vi "SEA-9811_ReceiverLoopback_FPGA.vi"() -> ()   [LabVIEW 2017]
doc: "This example demonstrates the SEA 9811 loopback mode. Please use the corresponding RT VI to operate this FPGA VI. \n\nCopyright (c) 2013-2019 S.E.A. Datentechnik GmbH, Germany"
uses:
  <vilib>/eio/EIOPropertyNode/EIOPropertyNode.xnode
  <vilib>/rvi/eio/common/nirviEmuTemplateMethod_errors.vi
  <vilib>/rvi/eio/common/nirviEmuTemplatePropertyGet_errors.vi
  <vilib>/rvi/eio/common/nirviEmuTemplatePropertyGet_noerrors.vi
  <vilib>/rvi/eio/common/nirviEmuTemplatePropertySet_errors.vi
  <vilib>/rvi/eio/common/nirviEmuTemplatePropertySet_noerrors.vi
  <vilib>/eio/EIOMethodNode/EIOMethodNode.xnode
  <vilib>/eio/EIONode/EIONode.xnode
panel:
  in  "Rx ConfigData":u16 format="%04x"
  in  "Read Rx Data":bool
  in  "Write Rx SimData":bool
  out "Rx Status Register":u16=255 format="%016b"
  out "CH7":u32 format="%08x"
  out "CH6":u32 format="%08x"
  out "CH5":u32 format="%08x"
  out "CH4":u32 format="%08x"
  out "CH3":u32 format="%08x"
  out "CH2":u32 format="%08x"
  out "CH1":u32 format="%08x"
  out "CH0":u32 format="%08x"
  in  "Rx Sim Data":u32=2271560481 format="%.0x"
  in  "stop":bool
  # "Please refer to VI description for instructions!"
  # "Note: \n\nThe transmitter doesn't send data in the bit order set in the control,\nbut rather changes the bit order when transmitting data. \nThe receiver changes the bit order back before outputting it,\nso that the original bit order is restored and the sent data\nequals the data received.\n\nThe Loopback transmitter DOES NOT change the data when transmitting. Therefore, in this FPGA VI the transmitted data does not equal the data received. Please refer to the real-time VI of this example to see how the data must be reversed to receive the same data at the receiver(s)."
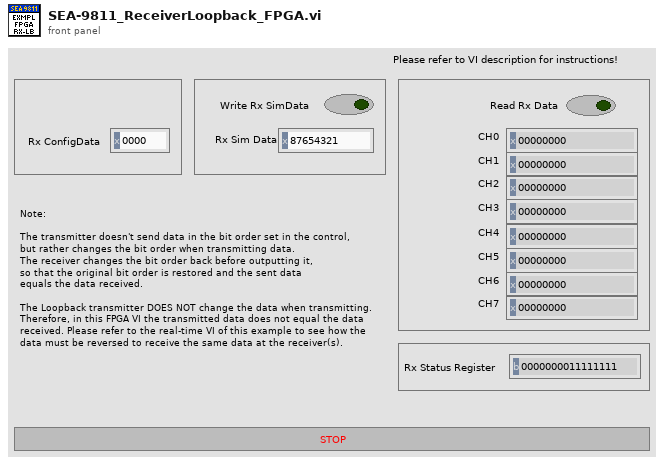
[diagram p1: front panel]
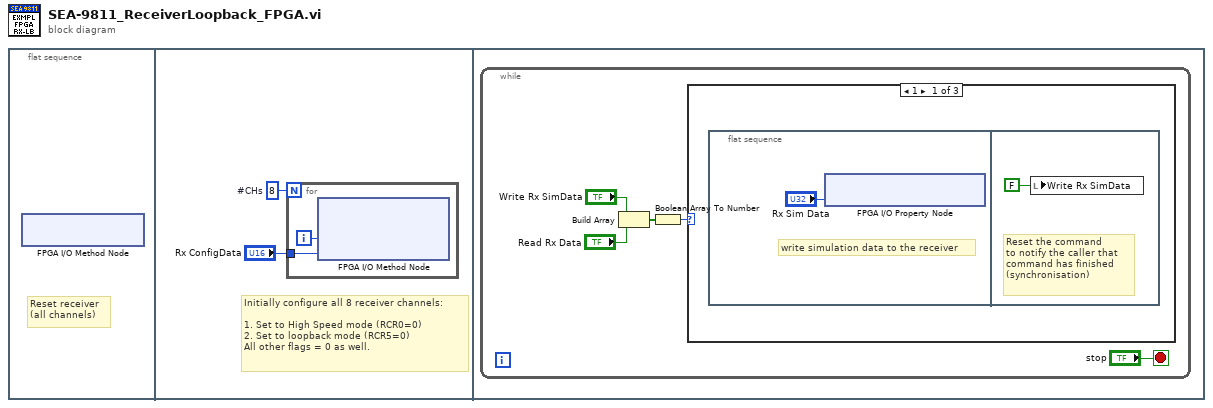
[diagram p0: block diagram]
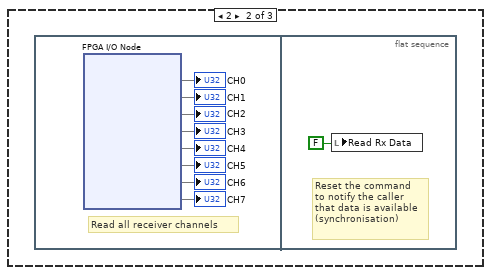
[diagram p2: hidden frame]
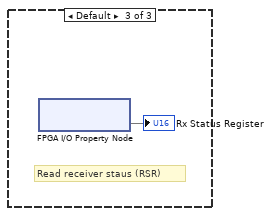
[diagram p3: hidden frame]
diagram:
  n1 = flat-sequence {
    frame #0 {
      # "Reset receiver\n(all channels)"
      n2 = xnode "FPGA I/O Method Node"() -> ()  [unwired: 1 in, 1 out]
    }
    frame #1 {
      w2 = 8  # #CHs
      # "Initially configure all 8 receiver channels: \n\n1. Set to High Speed mode (RCR0=0)\n2. Set to loopback mode (RCR5=0)\nAll other flags = 0 as well."
      n3 = for {
        N: w2 -> [_]
        tunnel: "Rx ConfigData" -> [w4]
        i -> [w3]
        n4 = xnode "FPGA I/O Method Node"("Channel Number"=w3, "Control Register"=w4) -> ()  [unwired: 1 in, 1 out]
      }
    }
    frame #2 {
      n5 = while {
        stop <- "stop" stop-if-true
        n6 = Build Array("Write Rx SimData", "Read Rx Data") -> (w6:bool[])
        n7 = Boolean Array To Number(Boolean array=w6) -> (number=w5:u8)
        n8 = case shown="1" w5 {
          frame 1 {
            n9 = flat-sequence {
              frame #0 {
                # "write simulation data to the receiver"
                n10 = xnode "FPGA I/O Property Node"("Rx SimData HighSpeed"="Rx Sim Data") -> ()  [unwired: 1 in, 1 out]
              }
              frame #1 {
                # "Reset the command\nto notify the caller that\ncommand has finished\n(synchronisation)"
                n11 = local write "Write Rx SimData"(FALSE ("Write SimData")) -> ()
              }
            }
          }
          frame 2 {
            n12 = flat-sequence {
              frame #0 {
                # "Read all receiver channels"
                n13 = xnode "FPGA I/O Node"() -> ("Mod1/Rx0"=→"CH0", "Mod1/Rx1"=→"CH1", "Mod1/Rx2"=→"CH2", "Mod1/Rx3"=→"CH3", "Mod1/Rx4"=→"CH4", "Mod1/Rx5"=→"CH5", "Mod1/Rx6"=→"CH6", "Mod1/Rx7"=→"CH7")  [unwired: 8 in, 8 out]
              }
              frame #1 {
                # "Reset the command\nto notify the caller\nthat data is available\n(synchronisation)"
                n14 = local write "Read Rx Data"(FALSE ("Read Rx Data")) -> ()
              }
            }
          }
          frame Default {
            # "Read receiver staus (RSR)"
            n15 = xnode "FPGA I/O Property Node"() -> ("Rx Status"=→"Rx Status Register")  [unwired: 1 in, 1 out]
          }
        }
      }
    }
  }
